vi "draw_image.vi"(8 "File Path":path=path "C:/Users/Antonio Costanzo/Desktop/U16 Tiff/U16 Tiff/sgf.jpg", 9 "Color":bool, 10 "M":i32, 11 "max":i16) -> (1 "Array":u16[](array[numeric]), 3 "Image out":T1(plugin-control))   [LabVIEW 2017]
panel:
  out "output array":u8[](array[numeric])
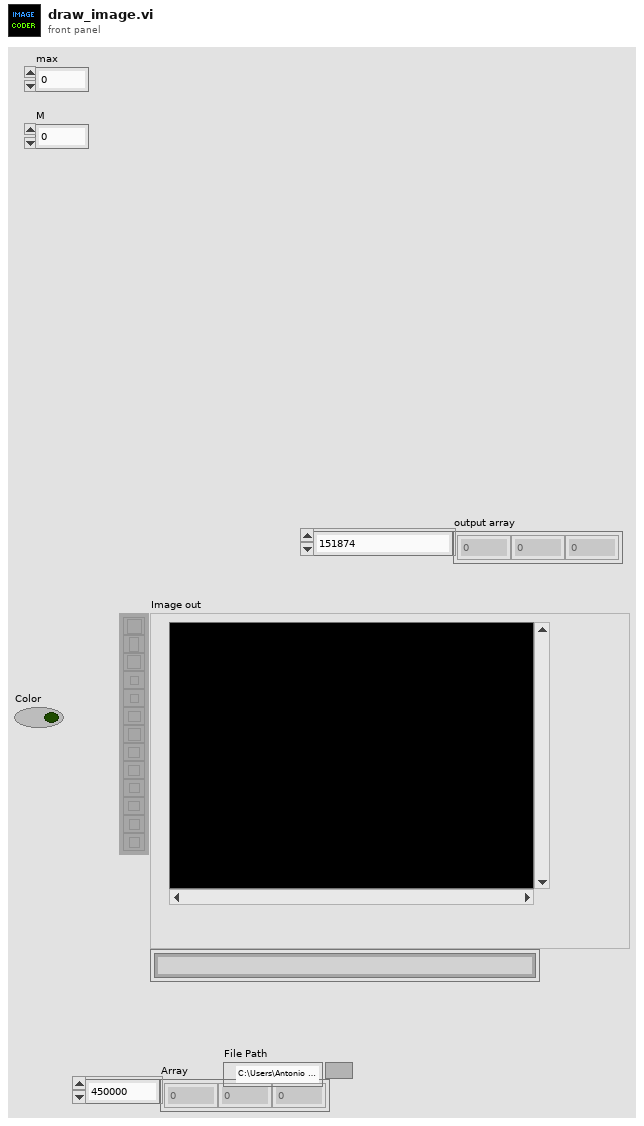
[diagram p1: front panel]
types:
  T1 = typedef "IMAQ Image.ctl" = refnum<image>
  T2 = typedef "Image Type" = u32
  T3 = typedef "imagedata.ctl" = cluster{"image type":i32, "image depth":i32, "image":u8[], "mask":u8[], "colors":u32[], "Rectangle":cluster{"left":i16, "top":i16, "right":i16, "bottom":i16}}
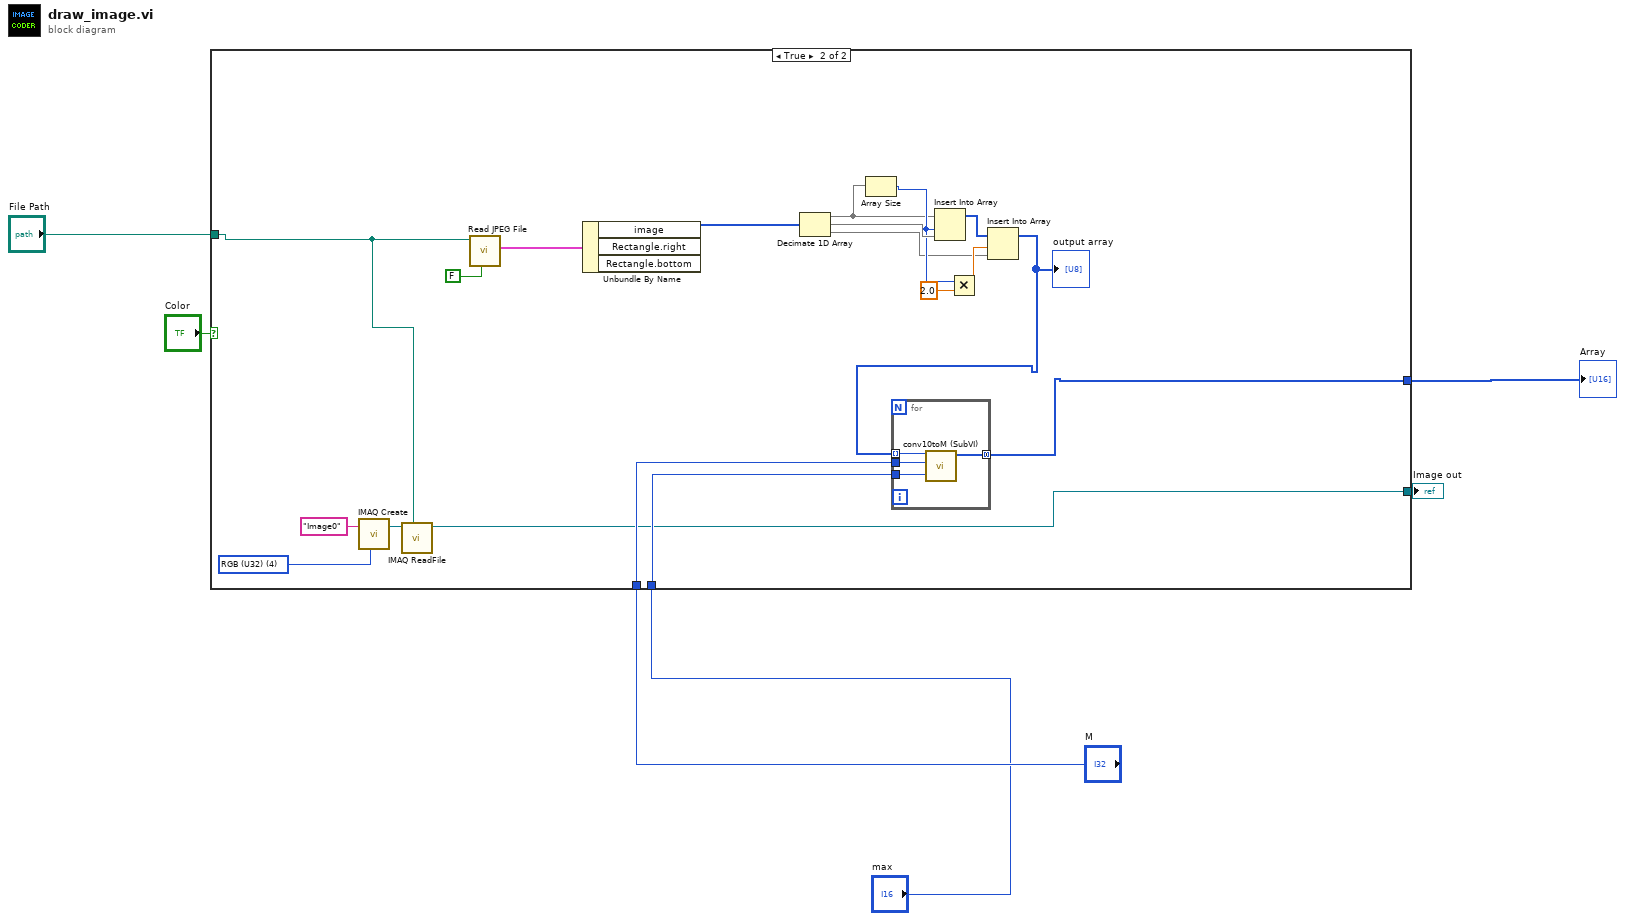
[diagram p0: block diagram]
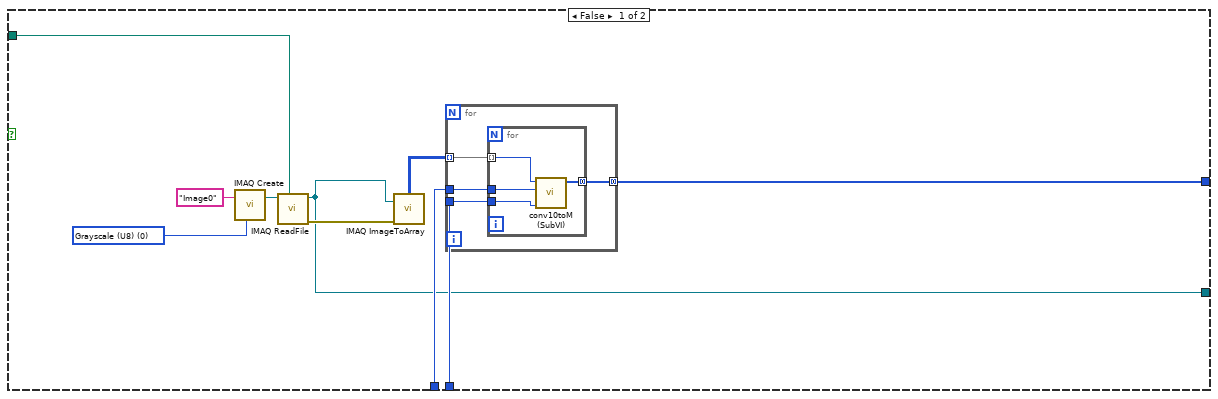
[diagram p2: hidden frame]
diagram:
  n1 = case shown="True" "Color" {
    tunnel: "M" -> [w16 w29]
    tunnel: [w15 w30] -> w5
    tunnel: "max" -> [w14 w28]
    tunnel: "File Path" -> [w8 w32]
    tunnel: [w7 w27] -> w1
    frame False {
      w12 = T2 0 items=["Grayscale (U8)", "Grayscale (I16)", "Grayscale (SGL)", "Complex (CSG)", "RGB (U32)", "HSL (U32)", "RGB (U64)"] ("Image Type")
      n2 = call "IMAQ Create"("Image Name"="Image0", "Image Type"=w12) -> ("New Image"=w9:T1)  [unwired: 3 in, 1 out]
      n3 = call "IMAQ ReadFile"("File Path"=w8, "Image"=w9) -> ("error out"=w11:errorcluster, "Image Out"=w7:T1)  [unwired: 5 in, 3 out]
      n4 = call "IMAQ ImageToArray"("error in (no error)"=w11, "Image"=w7) -> ("Image Pixels (U8)"=w13:u8[][])  [unwired: 2 in, 4 out]
      n5 = for {
        tunnel: w13 -> [w20] mode=indexing
        tunnel: [w19] -> w15 mode=concatenating
        tunnel: w16 -> [w18]
        tunnel: w14 -> [w17]
        n6 = for {
          tunnel: w20 -> [w24] mode=indexing
          tunnel: [w23] -> w19 mode=concatenating
          tunnel: w18 -> [w22]
          tunnel: w17 -> [w21]
          n7 = call "conv10toM (SubVI).vi"("max"=w21, "Base"=w22, "Input"=w24) -> ("Array"=w23:u8[])  [unwired: 8 in]
        }
      }
    }
    frame True {
      w38 = T2 4 items=["Grayscale (U8)", "Grayscale (I16)", "Grayscale (SGL)", "Complex (CSG)", "RGB (U32)", "HSL (U32)", "RGB (U64)"] ("Image Type")
      n8 = call "IMAQ Create"("Image Name"="Image0", "Image Type"=w38) -> ("New Image"=w40:T1)  [unwired: 3 in, 1 out]
      n9 = call "IMAQ ReadFile"("File Path"=w32, "Image"=w40) -> ("Image Out"=w27:T1)  [unwired: 5 in, 4 out]
      n10 = call <vilib>:"Read JPEG File.vi"("use 8 bit color table"=FALSE, "path to JPEG file"=w32) -> ("image data"=w41:T3)  [unwired: 7 in, 2 out]
      n11 = Unbundle By Name(w41) -> ("image"=w42:u8[])  [unwired: 2 out]
      n12 = Decimate 1D Array(w42) -> (w26:u8[], w35:u8[], w25:u8[])
      n13 = Array Size(array=w26) -> (size(s)=w34:i32)
      n14 = Insert Into Array(array=w26, index=w34, new element=w35) -> (w37:u8[])
      n15 = Multiply(x=w34, y=2.0) -> (x*y=w33:dbl)
      n16 = Insert Into Array(array=w37, index=w33, new element=w25) -> (w31:u8[])
      "output array" <- w31
      n17 = for {
        tunnel: [w47] -> w30 mode=concatenating
        tunnel: w29 -> [w46]
        tunnel: w28 -> [w45]
        tunnel: w31 -> [w44] mode=indexing
        n18 = call "conv10toM (SubVI).vi"("max"=w45, "Base"=w46, "Input"=w44) -> ("Array"=w47:u8[])  [unwired: 8 in]
      }
    }
  }
  "Array" <- w5
  "Image out" <- w1
